vi "CleanString.vi"(7 "Input":string) -> (1 "Cleaned":string)   [LabVIEW 2024]
panel:
  # "Cleans strings for special characters"
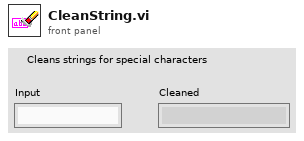
[diagram p1: front panel]
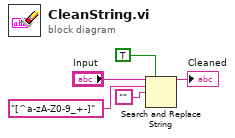
[diagram p0: block diagram]
diagram:
  n1 = Search and Replace String(replace all?=TRUE ("replace all? (F)"), input string="Input", search string="[^a-zA-Z0-9_+-]", replace string="") -> (result string=→"Cleaned":string)  [unwired: 4 in, 3 out]
